vi "Command.vi"(7 "Serial Device Brand":T1, 9 "Param 2":string, 10 "Param 1":string, 11 "Command":T2) -> (3 "Command to send":string)   [LabVIEW 2020, in "Serial device.lvclass"]
doc: "Template de un comando"
uses:
  Serial device.lvclass
  Controles/Command combobox.ctl
  Controles/Brand combobox.ctl
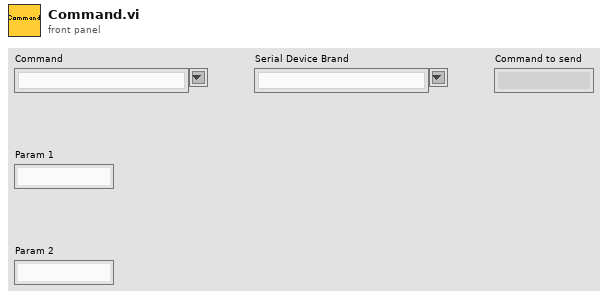
[diagram p1: front panel]
types:
  T1 = typedef "Serial device.lvclass/Brand combobox.ctl" = string
  T2 = typedef "Serial device.lvclass/Command combobox.ctl" = string
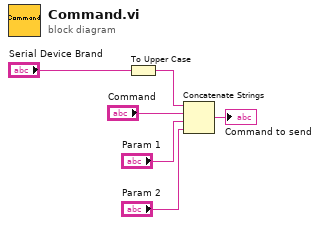
[diagram p0: block diagram]
diagram:
  n1 = To Upper Case(1:"Serial Device Brand") -> (0:w6:T1)
  n2 = Concatenate Strings(w6, "Command", "Param 1", "Param 2") -> (→"Command to send":string)
